vi "test Loopback_Complex.vi"(8 "error in":errorcluster, 11 "TestCase in":refnum<class "SingleCore.lvclass">) -> (0 "error out":errorcluster, 3 "TestCase out":refnum<class "SingleCore.lvclass">)   [LabVIEW 2020, in "SingleCore.lvclass"]
uses:
  SingleCore.lvclass
  C:/Git/niveristand-custom-device-testing-tools/VeriStandTestCase/VeriStandTestCase.lvclass
  4b06c685-66bb-4135-9ad1-d89a50a95502.vi
  <vilib>/numeric/Random Number (Range) DBL.vi
  4cc353ea-8eb2-4b69-8f0e-bf7f0ec9a5d6.vi
  <vilib>/NI VeriStand/Execution/Workspace/NI VeriStand - Set Multiple Channel Values.vi
  <vilib>/NI VeriStand/Execution/Workspace/NI VeriStand - Get Multiple Channel Values.vi
  <vilib>/addons/_JKI Toolkits/VI Tester/TestCase.llb/TestCase.lvclass
  niveristand-custom-device-testing-tools/VeriStandTestCase/VeriStandTestCase.lvclass
  <vilib>/NI VeriStand/Execution/Workspace/NI_VS Workspace ExecutionAPI.lvlib
  C:/Program Files (x86)/National Instruments/LabVIEW 2020/vi.lib/addons/_JKI Toolkits/VI Tester/TestCase.llb/TestCase.lvclass
  C:/Git/niveristand-ballard-arinc429-custom-device/Source/Custom Device Support/Tests/System/Loopback/SingleCore (P2--P3)/SingleCore.lvclass
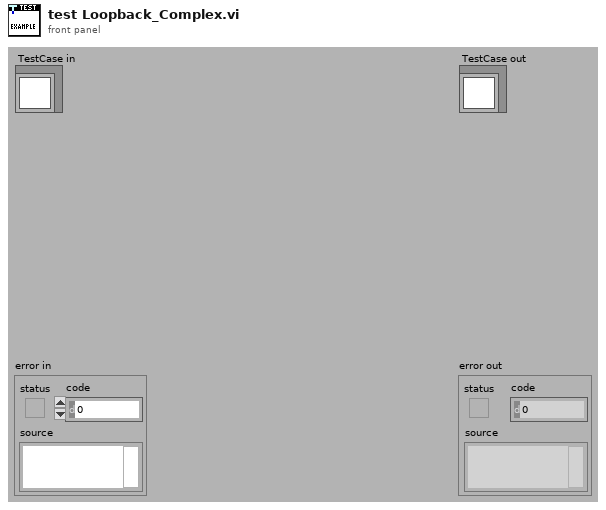
[diagram p1: front panel]
types:
  T1 = typedef "NI_VS Workspace ExecutionAPI.lvlib/WorkspaceAPI.ctl" = refnum<k24>
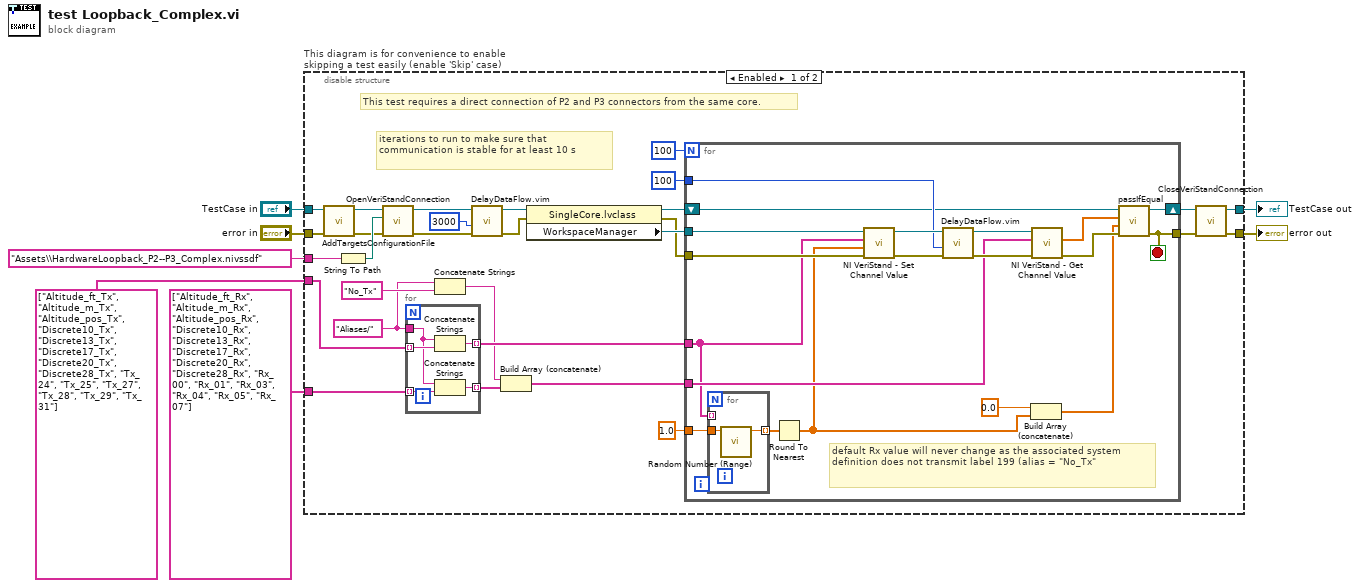
[diagram p0: block diagram]
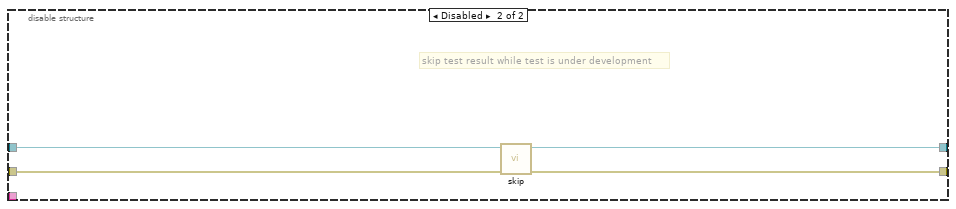
[diagram p2: hidden frame]
diagram:
  n1 = disable-structure "This diagram is for convenience to enable skipping a test easily (enable 'Skip' case)" shown="Enabled" {
    disable-tunnel: "TestCase in" -> [w35 w64]
    disable-tunnel: [w25 w62] -> w4
    disable-tunnel: [w24 w63] -> w6
    disable-tunnel: "error in" -> [w34 w61]
    disable-tunnel: "Assets\\HardwareLoopback_P2--P3_Complex.nivssdf" ("Channel") -> [w26 _]
    disable-tunnel: string[] ["Altitude_ft_Tx", "Altitude_m_Tx", "Altitude_pos_Tx", "Discrete10_Tx", "Discrete13_Tx", "Discrete17_Tx", "Discrete20_Tx", "Discrete28_Tx", "Tx_24", "Tx_25", "Tx_27", "Tx_28", "Tx_29", "Tx_31"] -> [w16 _]
    disable-tunnel: string[] ["Altitude_ft_Rx", "Altitude_m_Rx", "Altitude_pos_Rx", "Discrete10_Rx", "Discrete13_Rx", "Discrete17_Rx", "Discrete20_Rx", "Discrete28_Rx", "Rx_00", "Rx_01", "Rx_03", "Rx_04", "Rx_05", "Rx_07"] -> [w15 _]
    frame Enabled {
      w8 = "Aliases/" ("Channel")
      # "This test requires a direct connection of P2 and P3 connectors from the same core."
      # "iterations to run to make sure that communication is stable for at least 10 s"
      n2 = call "AddTargetsConfigurationFile.vi"("error in (no error)"=w34, "VeriStandTestCase in"=w35) -> ("error out"=w27:errorcluster, "VeriStandTestCase out"=w28:refnum<class "SingleCore.lvclass">)  [unwired: 8 in]
      n3 = String To Path(string=w26) -> (path=w29:path)
      n4 = call-dynamic "OpenVeriStandConnection.vi"("error in (no error)"=w27, "System Definition File"=w29, "VeriStand Test Case in"=w28) -> ("error out"=w31:errorcluster, "VeriStand Test Case out"=w33:refnum<class "SingleCore.lvclass">)  [unwired: 6 in, 1 out]
      n5 = for {
        tunnel: w8 -> [w38]
        tunnel: w16 -> [w40] mode=indexing
        tunnel: w15 -> [w39] mode=indexing
        tunnel: [w37] -> w14 mode=indexing
        tunnel: [w36] -> w12 mode=indexing
        n6 = Concatenate Strings(w38, w40) -> (w37:string)
        n7 = Concatenate Strings(w38, w39) -> (w36:string)
      }
      n8 = Concatenate Strings(w8, "No_Tx" ("Channel")) -> (w13:string)
      n9 = call "DelayDataFlow.vim"("value in"=w31, "milliseconds to wait"=u32 3000) -> ("value out"=w30:errorcluster)  [unwired: 2 in, 1 out]
      n10 = Build Array (concatenate)(w13, w12) -> (w11:string[])
      n11 = property class="SingleCore.lvclass"(reference=w33, error in=w30) -> (reference out=w19:refnum<class "SingleCore.lvclass">, error out=w20:errorcluster, "WorkspaceManager"=w23:T1)
      n12 = for {
        N: 100 -> [_]
        tunnel: w14 -> [w41]
        tunnel: w23 -> [w55]
        tunnel: u32 100 ("milliseconds to wait") -> [w54]
        tunnel: w20 -> [w53]
        tunnel: w11 -> [w47]
        shift-right: [w50] -> w18
        shift-left: w19 -> [w51]
        tunnel: [w48] -> w17
        tunnel: 1.0 ("upper bound (100)") -> [w43]
        stop <- w48 stop-if-true
        # "default Rx value will never change as the associated system definition does not transmit label 199 (alias = \"No_Tx\""
        n13 = for {
          tunnel: [w60] -> w45 mode=indexing
          tunnel: w43 -> [w59]
          tunnel: w41 -> [_] mode=indexing
          n14 = call-poly <vilib>:"Random Number (Range).vi"("upper bound (100)"=w59) -> ("number"=w60:dbl)  [unwired: 10 in]
        }
        n15 = Round To Nearest(number=w45) -> (nearest integer value=w42:dbl[])
        n16 = call-poly <vilib>:"NI VeriStand - Set Channel Value.vi"("error in (no error)"=w53, "Values"=w42, "Channels"=w41, "WorkspaceManager in"=w55) -> ("error out"=w57:errorcluster, "WorkspaceManager out"=w56:T1)  [unwired: 6 in]
        n17 = call "DelayDataFlow.vim"("value in"=w57, "milliseconds to wait"=w54) -> ("value out"=w58:errorcluster)  [unwired: 2 in, 1 out]
        n18 = Build Array (concatenate)(0.0 ("upper bound (100)"), w42) -> (w44:dbl[])
        n19 = call-poly <vilib>:"NI VeriStand - Get Channel Value.vi"("error in (no error)"=w58, "Channels"=w47, "WorkspaceManager in"=w56) -> ("error out"=w52:errorcluster, "Values"=w49:dbl[])  [unwired: 6 in, 1 out]
        n20 = call-dynamic "passIfEqual.vi"("error in (no error)"=w52, "y"=w44, "x"=w49, "TestCase in"=w51) -> ("error out"=w48:errorcluster, "TestCase out"=w50:refnum<class "SingleCore.lvclass">)  [unwired: 6 in]
      }
      n21 = call-dynamic "CloseVeriStandConnection.vi"("error in (no error)"=w17, "VeriStand Test Case in"=w18) -> ("error out"=w24:errorcluster, "VeriStand Test Case out"=w25:refnum<class "SingleCore.lvclass">)  [unwired: 8 in]
    }
    frame Disabled {
      # "skip test result while test is under development"
      n22 = call <vilib>:"skip.vi"("error in (no error)"=w61, "TestCase in"=w64) -> ("error out"=w63:errorcluster, "TestCase out"=w62:refnum<class "SingleCore.lvclass">)  [unwired: 8 in]
    }
  }
  "error out" <- w6
  "TestCase out" <- w4
